vi "Hardware-HHScope-Host.vi"() -> ()   [LabVIEW 2016]
uses:
  <vilib>/Powertrain Controls/Device Drivers/DCM/HH/FPGA/Capture Event.ctl
  <vilib>/Powertrain Controls/Device Drivers/DCM/HH/FPGA/DCM - FPGA - HH.lvlib
panel:
  in  "ScopeEvent":u8(ring) items=["Unused", "Injector A1", "Injector A2", "Injector A3", "Injector A4", "Injector A5", "Injector A6", "Injector A7", "Injector A8/PumpA", "Injector B1", "Injector B2", "Injector B3", "Injector B4", "Injector B5", "Injector B6", "Injector B7", "Injector B8/PumpB", "Diff IO 1", "Diff IO 2", "Diff IO 3", "Diff IO 4", "Diff IO 5", "Diff IO 6", "Diff IO 7", "Diff IO 8", "Aux 1", "Aux 2", "Aux 3", "Aux 4", "Aux 5", "Aux 6", "Aux 7", "Aux 8", "User OS"]
  in  "_HHScopeEvent":T1
  in  "Capture":bool caption="ScopeEnable"
  in  "Length":sgl=0.01 caption="[s]" min=0 max=0.055 format="%#_6p"
  out "_HH Scope":sgl[][](graph)
  out "Data":sgl[][](array[numeric])
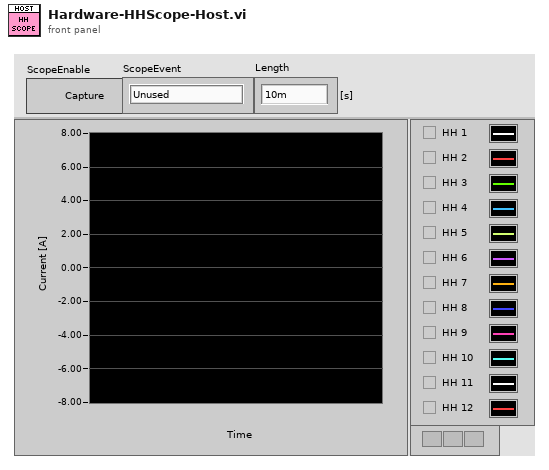
[diagram p1: front panel]
types:
  T1 = typedef "DCM - FPGA - HH.lvlib/Capture Event.ctl" = enum8{"Unused", "HH 1", "HH 2", "HH 3", "HH 4", "HH 5", "HH 6", "HH 7", "HH 8", "HH 9", "HH 10", "HH 11", "HH 12"}
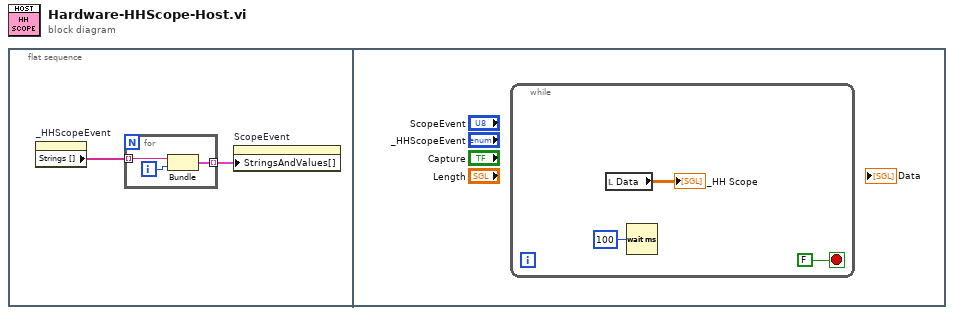
[diagram p0: block diagram]
diagram:
  n1 = flat-sequence {
    frame #0 {
      n2 = property on="_HHScopeEvent" class="Enum (strict)"() -> ("Strings []"=w1:string[])  [unwired: 2 in, 2 out]
      n3 = for {
        tunnel: w1 -> [w5] mode=indexing
        tunnel: [w3] -> w2 mode=indexing
        i -> [w4]
        n4 = Bundle(w5, w4) -> (w3:cluster{string, i32})  [unwired: 1 in]
      }
      n5 = property on="ScopeEvent" class="Ring (strict)"("StringsAndValues[]"=w2) -> ()  [unwired: 2 in, 2 out]
    }
    frame #1 {
      n6 = while {
        stop <- FALSE stop-if-true
        n7 = local read "Data"() -> (→"_HH Scope":sgl[][])
        n8 = Wait (ms)(milliseconds to wait=u32 100) -> ()  [unwired: 1 out]
      }
    }
  }
